vi "QI radial profile calculate.vi"(6 "ROI array":u8[][](array[numeric]), 7 "num":i32, 9 "Yr":dbl, 10 "Xr":dbl, 11 "r":dbl) -> (1 "mean3":dbl, 2 "mean2":dbl, 3 "mean1":dbl, 5 "mean4":dbl)   [LabVIEW 2017]
uses:
  <vilib>/Analysis/baseanly.llb/Mean (DBL).vi
  <vilib>/Analysis/NI_AALBase.lvlib
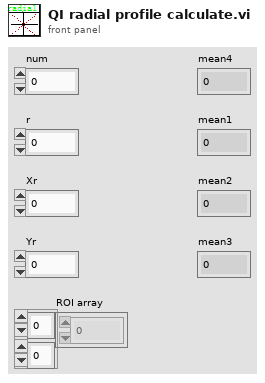
[diagram p1: front panel]
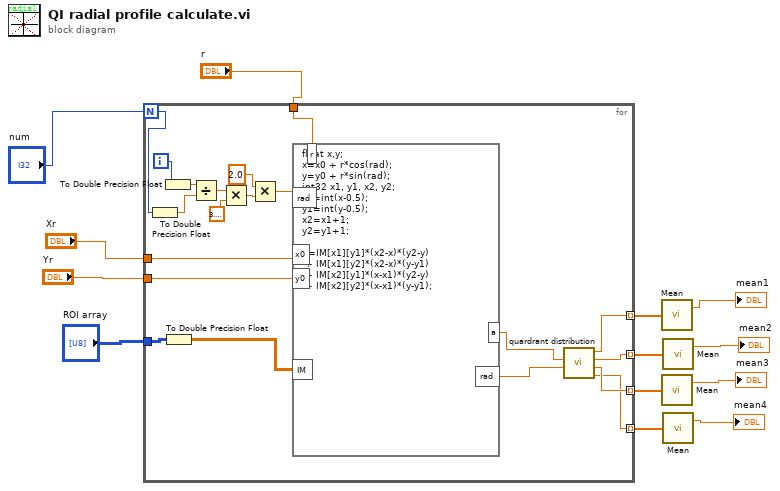
[diagram p0: block diagram]
diagram:
  n1 = for "For循环" {
    N: "num" -> [w26]
    tunnel: "Xr" -> [w29]
    tunnel: "Yr" -> [w28]
    tunnel: "r" -> [w23]
    tunnel: "ROI array" -> [w22]
    tunnel: [w17] -> w5 mode=indexing
    tunnel: [w16] -> w7 mode=indexing
    tunnel: [w15] -> w8 mode=indexing
    tunnel: [w14] -> w9 mode=indexing
    i -> [w27]
    n2 = To Double Precision Float(number=w26) -> (double precision float=w21:dbl)
    n3 = To Double Precision Float(number=w27) -> (double precision float=w30:dbl)
    n4 = To Double Precision Float(number=w22) -> (double precision float=w20:dbl[][])
    n5 = Divide(x=w30, y=w21) -> (x/y=w33:dbl)
    n6 = Multiply(x=w33, y=3.141592653589793) -> (x*y=w32:dbl)
    n7 = Multiply(x=2.0, y=w32) -> (x*y=w25:dbl)
    n8 = formula code="float x,y;\nx=x0 + r*cos(rad);\ny=y0 + r*sin(rad);\nint32 x1, y1, x2, y2;\nx1=int(x-0.5);\ny1=int(y-0.5);\nx2=x1+1;\ny2=y1+1;\n\na=IM[x1][y1]*(x2-x)*(y2-y)\n + IM[x1][y2]*(x2-x)*(y-y1)\n + IM[x2][y1]*(x-x1)*(y2-y)\n + IM[x2][y2]*(x-x1)*(y-y1);"("x0"=w29, "y0"=w28, "rad"=w25, "r"=w23, "IM"=w20) -> ("rad"=w18:dbl, "a"=w19:dbl)
    n9 = call "quardrant distribution.vi"("rad"=w18, "input radial point"=w19) -> ("quardrant 4"=w14:dbl, "quardrant 3"=w15:dbl, "quardrant 2"=w16:dbl, "quardrant 1"=w17:dbl)  [unwired: 6 in]
  }
  n10 = call-poly <vilib>:"Mean.vi"("X"=w5) -> ("mean"=→"mean1":dbl)  [unwired: 1 out]
  n11 = call-poly <vilib>:"Mean.vi"("X"=w8) -> ("mean"=→"mean3":dbl)  [unwired: 1 out]
  n12 = call-poly <vilib>:"Mean.vi"("X"=w7) -> ("mean"=→"mean2":dbl)  [unwired: 1 out]
  n13 = call-poly <vilib>:"Mean.vi"("X"=w9) -> ("mean"=→"mean4":dbl)  [unwired: 1 out]
